vi "Caller's VI Reference.vi"(0 "error in (no error)":errorcluster) -> (5 "error out":errorcluster, 6 "Caller's VI Reference":refnum<vi>)   [LabVIEW 2017, in "TagDB RefManager.lvlib"]
uses:
  TagDB RefManager.lvlib
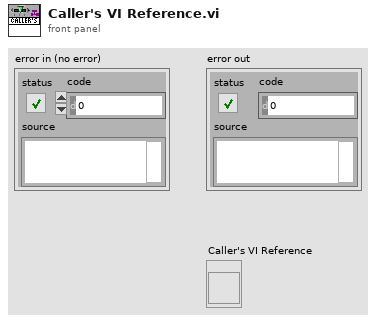
[diagram p1: front panel]
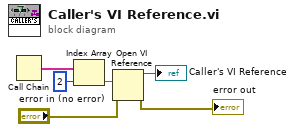
[diagram p0: block diagram]
diagram:
  n1 = Call Chain() -> (call chain=w5:string[])
  n2 = Index Array(array=w5, index=2) -> (element=w4:string)
  n3 = Open VI Reference(vi path=w4, error in (no error)="error in (no error)") -> (vi reference=→"Caller's VI Reference":refnum<vi>, error out=→"error out":errorcluster)  [unwired: 4 in]
